vi "Get Details from Error XML.vi"(11 "Error XML":string) -> (3 "Details":string)   [LabVIEW 2015, in "NI_Azure_Core.lvlib"]
uses:
  NI_Azure_Core.lvlib
  XML Parsing/NI_Azure_XML Parsing.lvlib
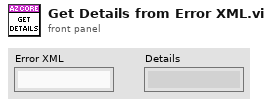
[diagram p1: front panel]
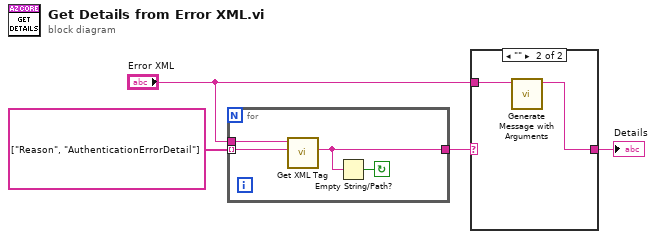
[diagram p0: block diagram]
diagram:
  n1 = for {
    tunnel: string[] ["Reason", "AuthenticationErrorDetail"] -> [w8] mode=indexing
    tunnel: "Error XML" -> [w7]
    tunnel: [w5] -> w3
    stop <- w6 continue-if-true
    n2 = call "Get XML Tag.vi"("Tag name"=w8, "XML String in"=w7) -> ("Tag value"=w5:string)  [unwired: 5 in, 4 out]
    n3 = Empty String/Path?(string/path=w5) -> (empty?=w6:bool)
  }
  n4 = case shown="\"\"" w3 {
    selector: w3 -> [w9 _]
    tunnel: "Error XML" -> [_ w11]
    tunnel: [w9 w10] -> w1
    frame Default {
    }
    frame "" {
      n5 = call "Generate Message with Arguments.vi"("XML String"=w11) -> ("Message with Arguments"=w10:string)  [unwired: 10 in]
    }
  }
  "Details" <- w1
